vi "emi_Tab visibility by name.vi"(0 "reference":refnum<vi>, 7 "Visibil(T)":bool=TRUE, 11 "error in (no error)":errorcluster, 12 "Tab name(\"Debug\")":string="Debug") -> (4 "reference out":refnum<vi>, 15 "error out":errorcluster)   [LabVIEW 2011]
doc: "Setting a tab visible or hidden based on name. \n\nOn Error: Do nothing"
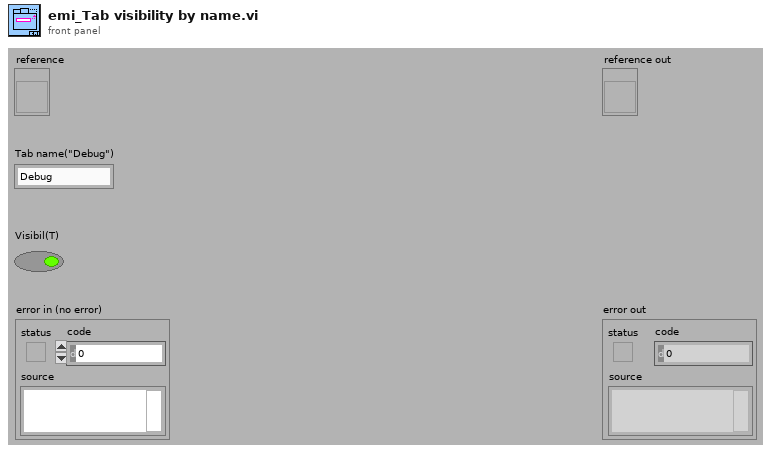
[diagram p1: front panel]
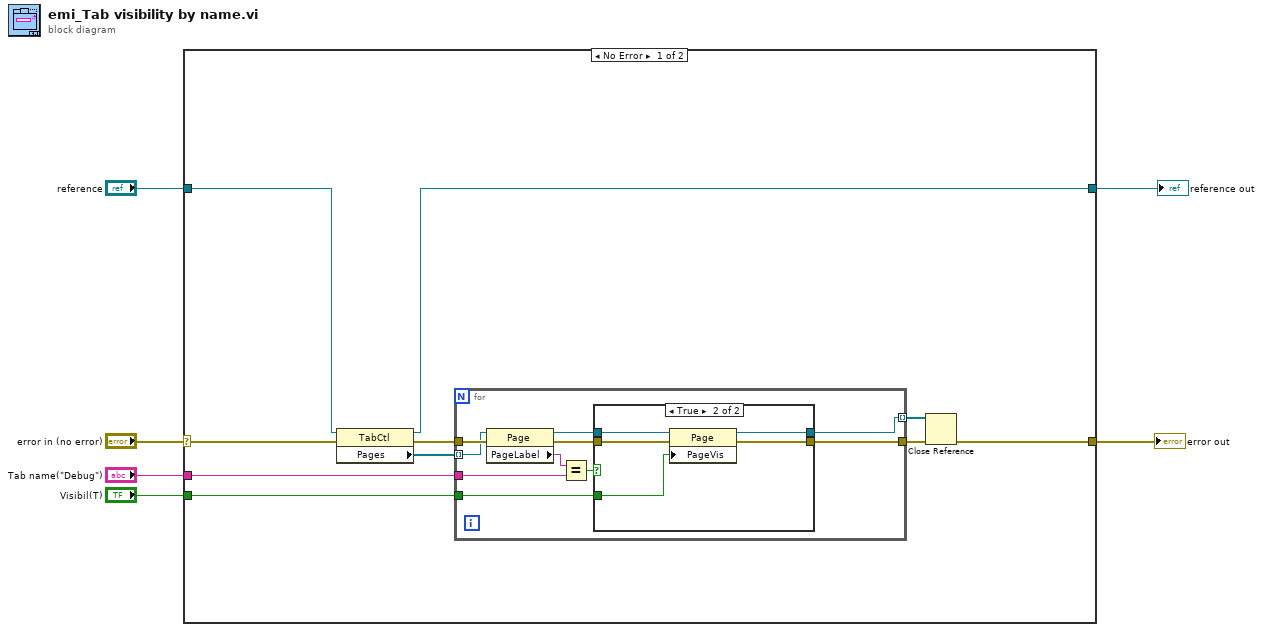
[diagram p0: block diagram]
diagram:
  n1 = case shown="No Error" "error in (no error)" {
    selector: "error in (no error)" -> [w15 w35]
    tunnel: [w10 w35] -> w5
    tunnel: "reference" -> [w16 w34]
    tunnel: [w14 w34] -> w3
    tunnel: "Tab name(\"Debug\")" -> [w8 _]
    tunnel: "Visibil(T)" -> [w7 _]
    frame No Error {
      n2 = property class="TabCtl"(reference=w16, error in=w15) -> (reference out=w14:refnum<vi>, error out=w12:errorcluster, "Pages"=w11:refnum<vi>[])
      n3 = for {
        tunnel: [w21] -> w13
        tunnel: w12 -> [w26]
        tunnel: w11 -> [w25] mode=indexing
        tunnel: [w19] -> w9 mode=indexing
        tunnel: w8 -> [w22]
        tunnel: w7 -> [w17]
        n4 = property class="Page"(reference=w25, error in=w26) -> (reference out=w18:refnum<vi>, error out=w20:errorcluster, "PageLabel"=w23:string)
        n5 = Equal?(x=w23, y=w22) -> (x = y?=w24:bool)
        n6 = case shown="True" w24 {
          tunnel: [w27 w30] -> w21
          tunnel: w20 -> [w27 w33]
          tunnel: [w28 w31] -> w19
          tunnel: w18 -> [w28 w32]
          tunnel: w17 -> [_ w29]
          frame False {
          }
          frame True {
            n7 = property class="Page"(reference=w32, error in=w33, "PageVis"=w29) -> (reference out=w31:refnum<vi>, error out=w30:errorcluster)
          }
        }
      }
      n8 = Close Reference(reference=w9, error in (no error)=w13) -> (error out=w10:errorcluster)
    }
    frame Error {
    }
  }
  "error out" <- w5
  "reference out" <- w3
